vi "Write File Header.vi"(8 "error in":errorcluster, 10 "File Header":string, 11 "File Actor in":refnum<class "File Actor.lvclass">) -> (0 "error out":errorcluster, 3 "File Actor out":refnum<class "File Actor.lvclass">)   [LabVIEW 2017, in "File Library.lvlib" / "File Actor.lvclass"]
uses:
  File Actor.lvclass
  File Actor.lvclass/File Actor.ctl
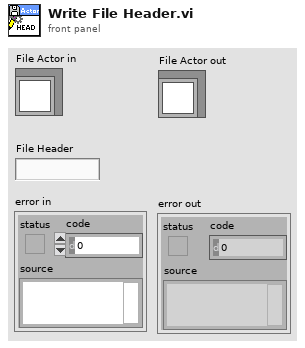
[diagram p1: front panel]
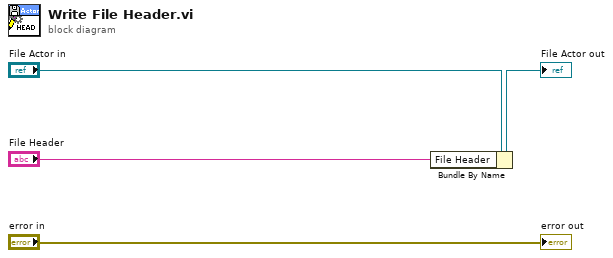
[diagram p0: block diagram]
diagram:
  n1 = Bundle By Name(cluster="File Actor in", "File Header"="File Header") -> (→"File Actor out":refnum<class "File Actor.lvclass">)
  "error out" <- "error in"
